vi "test15-StateBroadcast_Event.vi"(8 "error in (no error)":errorcluster, 11 "TestCase in":refnum<class "testcase-CSMGlobalLog.lvclass">) -> (0 "error out":errorcluster, 3 "TestCase out":refnum<class "testcase-CSMGlobalLog.lvclass">)   [LabVIEW 2017, in "testcase-CSMGlobalLog.lvclass"]
uses:
  testcase-CSMGlobalLog.lvclass
  testcase-CSMGlobalLog.lvclass/testcase-CSMGlobalLog.ctl
  src/user.lib/_NEVSTOP/Communicable State Machine(CSM)/_Support/Typedef/_CSM_GlobalLog_MSG.ctl
  src/user.lib/_NEVSTOP/Communicable State Machine(CSM)/_Support/Typedef/_CSM_Response Source Message.ctl
  src/user.lib/_NEVSTOP/Communicable State Machine(CSM)/_Support/Typedef/_CSM_GlobalLog_MSG_TYPE.ctl
  c0dc643a-0362-49fc-99f4-5251266ba5a0.vi
  src/user.lib/_NEVSTOP/Communicable State Machine(CSM)/_Support/GlobalEvent/GEvt-Generate with Rule Check.vi
  src/user.lib/_NEVSTOP/Communicable State Machine(CSM)/AdvanceAPI/CSM - Convert Error to Argument.vi
  src/user.lib/_NEVSTOP/Communicable State Machine(CSM)/AdvanceAPI/CSM - Make String Arguments Safe.vi
  src/user.lib/_NEVSTOP/Communicable State Machine(CSM)/AdvanceAPI/CSM - Keywords.vi
  src/user.lib/_NEVSTOP/Communicable State Machine(CSM)/_Support/GlobalEvent/Cache-GEvt Refs.vi
  src/user.lib/_NEVSTOP/Communicable State Machine(CSM)/_Support/GlobalEvent/LogFilter/LogFilter - Check.vi
  src/user.lib/_NEVSTOP/Communicable State Machine(CSM)/_Support/GlobalEvent/LogFilter/LogFilter.lvclass
  <vilib>/addons/_JKI Toolkits/VI Tester/TestCase.llb/TestCase.lvclass
  src/user.lib/_NEVSTOP/Communicable State Machine(CSM)/Communicable State Machine.lvlib
  C:/Program Files (x86)/National Instruments/LabVIEW 2017/vi.lib/addons/_JKI Toolkits/VI Tester/TestCase.llb/TestCase.lvclass
panel:
  out "String cache each loop":string
  out "error out 2":errorcluster
  out "Timed out":bool[](array[boolean])
  out "LoopCount":i32
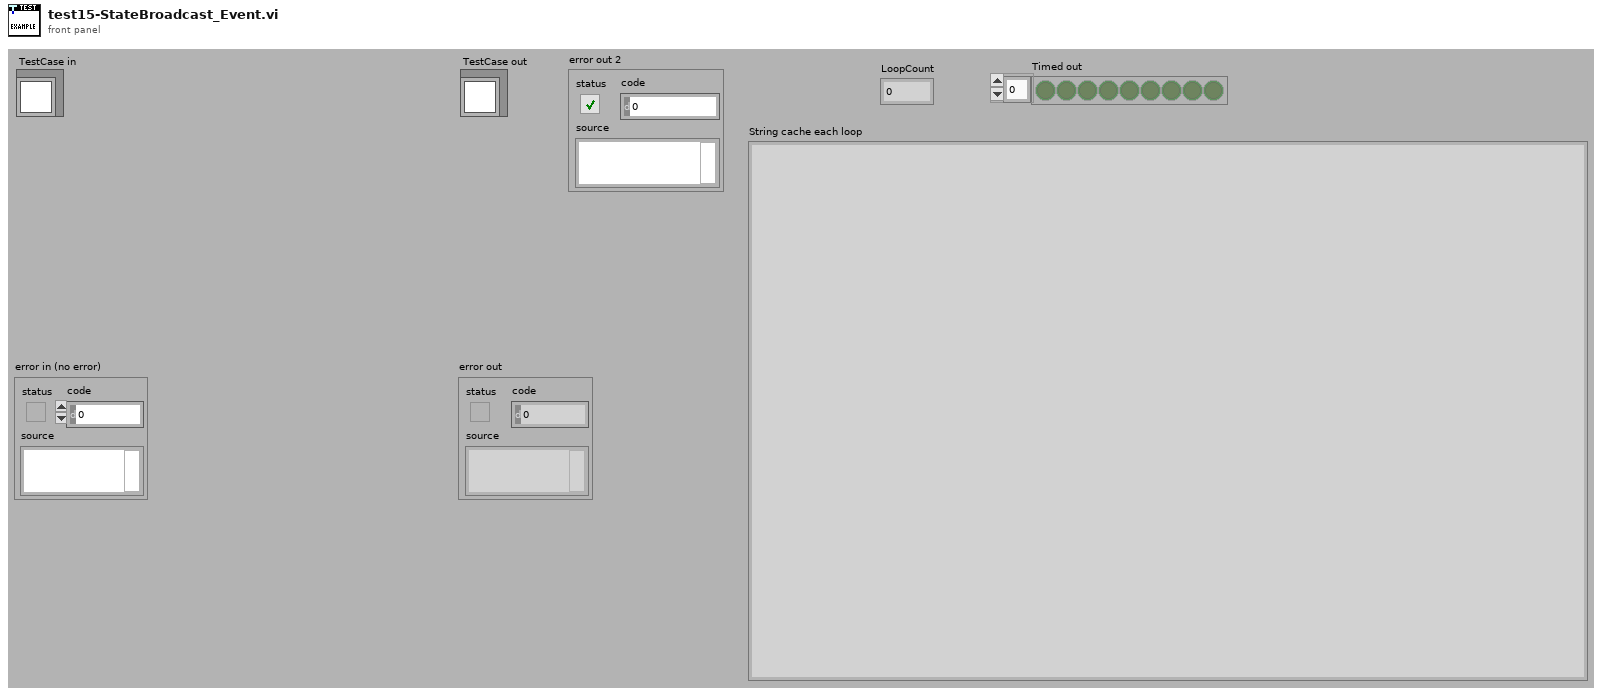
[diagram p1: front panel]
types:
  T1 = typedef "Communicable State Machine.lvlib/_CSM_GlobalLog_MSG.ctl" = cluster{"Name (\"\" to Use UUID)":string, "Current State":string, "Arguments":string, "Source Message":T2, "Source Module":string, "Complete(T)/Start(F)":bool, "LogType":T3, "Time Stamp":timestamp}
  T2 = typedef "Communicable State Machine.lvlib/_CSM_Response Source Message.ctl" = cluster{"‘State":string, "’Arguments":string, "’Error":errorcluster}
  T3 = typedef "Communicable State Machine.lvlib/_CSM_GlobalLog_MSG_TYPE.ctl" = enum16{"User Log", "State Change", "Status", "Interrupt", "Register", "Unregister", "Error Log", "Module Created", "Module Destroyed", "Async Message", "No-Rep Async Message", "Sync Message"}
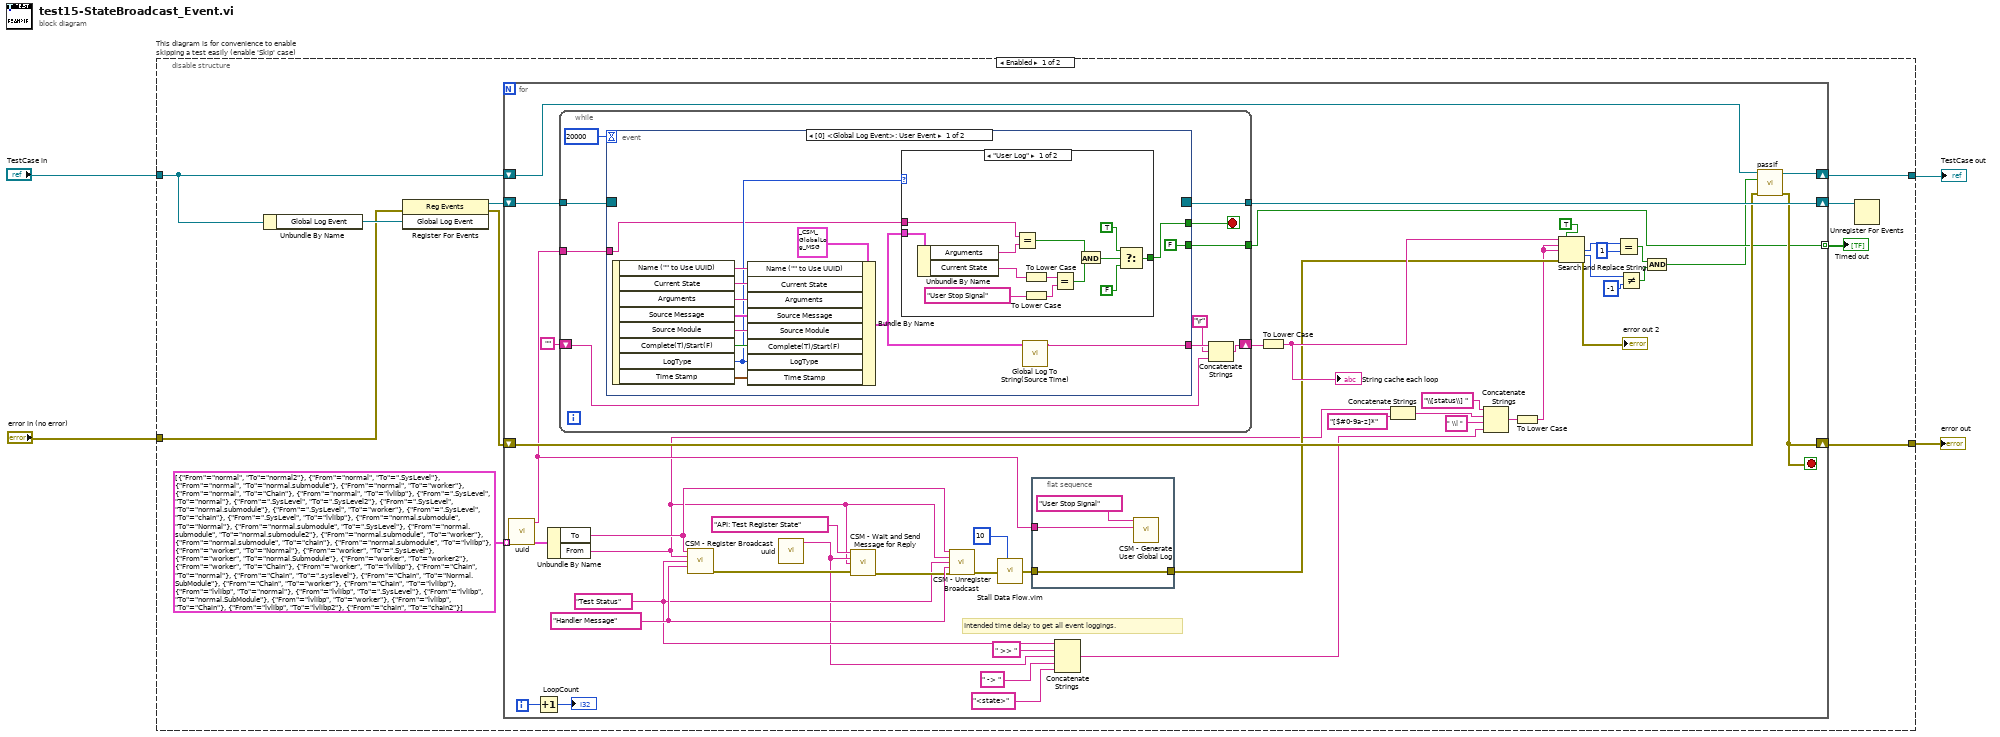
[diagram p0: block diagram]
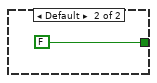
[diagram p2: hidden frame]
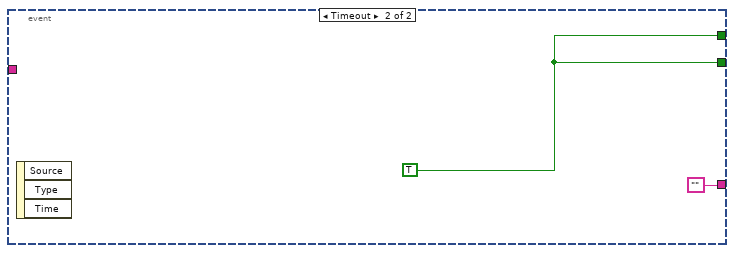
[diagram p3: hidden frame]
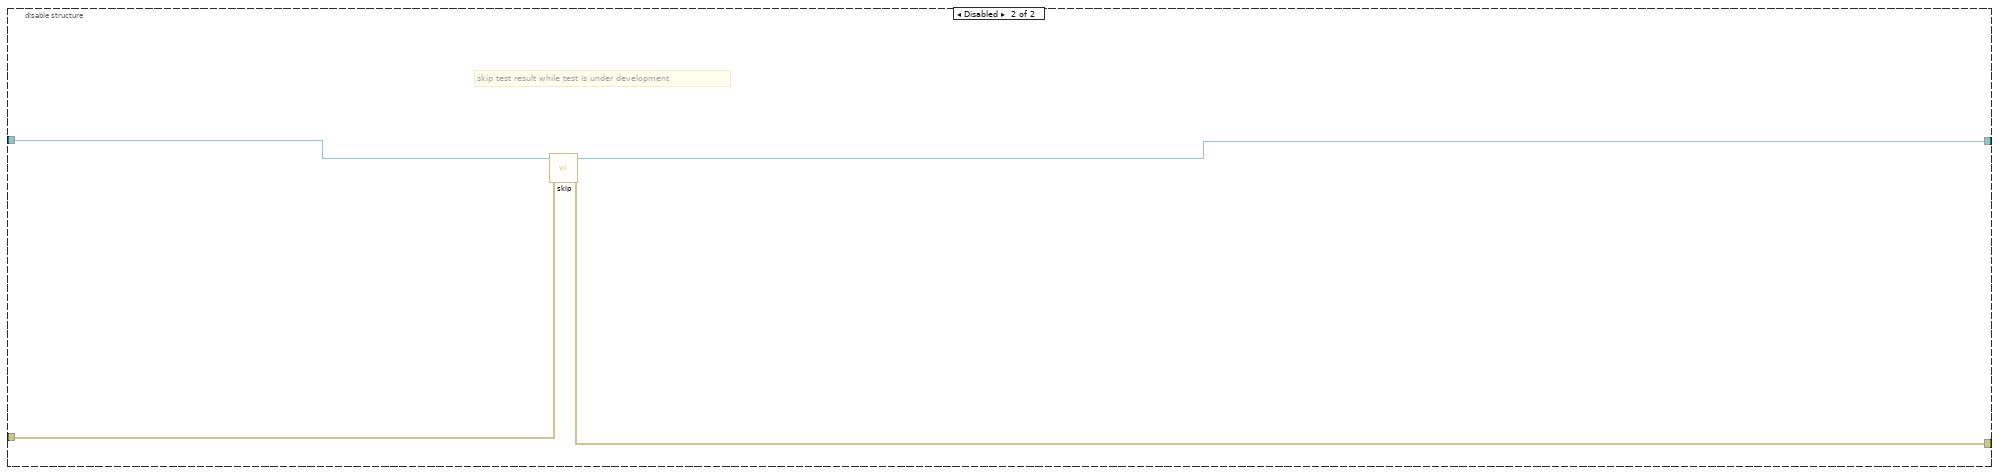
[diagram p4: hidden frame]
diagram:
  n1 = disable-structure "This diagram is for convenience to enable skipping a test easily (enable 'Skip' case)" shown="Enabled" {
    disable-tunnel: "TestCase in" -> [w9 w106]
    disable-tunnel: [w8 w104] -> w1
    disable-tunnel: [w7 w105] -> w3
    disable-tunnel: "error in (no error)" -> [w13 w103]
    frame Enabled {
      n2 = Unbundle By Name(w9) -> ("Global Log Event"=w14:refnum<user-event>)
      n3 = register-events(error in=w13, w14) -> (reference out=w12:refnum<event-registration>, error out=w10:errorcluster)  [unwired: 1 in]
      n4 = for {
        shift-right: [w58] -> w11
        shift-left: w12 -> [w59]
        shift-right: [w54] -> w7
        shift-left: w10 -> [w56]
        tunnel: cluster{"From":string, "To":string}[] [{"From"="normal", "To"="normal2"}, {"From"="normal", "To"=".SysLevel"}, {"From"="normal", "To"="normal.submodule"}, {"From"="normal", "To"="worker"}, {"From"="normal", "To"="Chain"}, {"From"="normal", "To"="lvlibp"}, {"From"=".SysLevel", "To"="normal"}, {"From"=".SysLevel", "To"=".SysLevel2"}, {"From"=".SysLevel", "To"="normal.submodule"}, {"From"=".SysLevel", "To"="worker"}, {"From"=".SysLevel", "To"="chain"}, {"From"=".SysLevel", "To"="lvlibp"}, {"From"="normal.submodule", "To"="Normal"}, {"From"="normal.submodule", "To"=".SysLevel"}, {"From"="normal.submodule", "To"="normal.submodule2"}, {"From"="normal.submodule", "To"="worker"}, {"From"="normal.submodule", "To"="chain"}, {"From"="normal.submodule", "To"="lvlibp"}, {"From"="worker", "To"="Normal"}, {"From"="worker", "To"=".SysLevel"}, {"From"="worker", "To"="normal.Submodule"}, {"From"="worker", "To"="worker2"}, {"From"="worker", "To"="Chain"}, {"From"="worker", "To"="lvlibp"}, {"From"="Chain", "To"="normal"}, {"From"="Chain", "To"=".syslevel"}, {"From"="Chain", "To"="Normal.SubModule"}, {"From"="Chain", "To"="worker"}, {"From"="Chain", "To"="lvlibp"}, {"From"="lvlibp", "To"="normal"}, {"From"="lvlibp", "To"=".SysLevel"}, {"From"="lvlibp", "To"="normal.SubModule"}, {"From"="lvlibp", "To"="worker"}, {"From"="lvlibp", "To"="Chain"}, {"From"="lvlibp", "To"="lvlibp2"}, {"From"="chain", "To"="chain2"}] -> [w31] mode=indexing
        shift-right: [w57] -> w8
        shift-left: w9 -> [w53]
        tunnel: [w37] -> w5 mode=indexing
        i -> [w42]
        stop <- w54 stop-if-true
        w36 = "Handler Message" ("API (If \"\", Same as Trigger)")
        w27 = "Test Status" ("Trigger")
        # "Intended time delay to get all event loggings."
        n5 = call "uuid.vi"() -> ("UUID"=w43:string)  [unwired: 11 in]
        n6 = Increment(x=w42) -> (x+1=→"LoopCount":i32)
        n7 = Unbundle By Name(w31) -> ("To"=w18:string, "From"=w17:string)
        n8 = while {
          tunnel: w59 -> [w72]
          tunnel: [w71] -> w58
          shift-right: [w63] -> w38
          shift-left: "" -> [w66]
          tunnel: w43 -> [w68]
          tunnel: [w67] -> w37
          stop <- w70 stop-if-true
          n9 = event shown="[0] <Global Log Event>: User Event" {
            selector: w72 -> [_ _]
            dyn-events: [_ _] -> w71
            timeout: 20000 -> [_ _]
            tunnel: [w73 ""] -> w65
            tunnel: [w75 w102] -> w70
            tunnel: w68 -> [w76 _]
            tunnel: [FALSE ("Stop") w102] -> w67
            event User Event {
              n10 = event-data() -> ("Name (\"\" to Use UUID)"=w85:string, "Current State"=w84:string, "Arguments"=w83:string, "Source Message"=w82:T2, "Source Module"=w81:string, "Complete(T)/Start(F)"=w80:bool, "LogType"=w77:T3, "Time Stamp"=w79:timestamp)  [unwired: 1 in]
              n11 = Bundle By Name(cluster=T1 {"Name (\"\" to Use UUID)"="", "Current State"="", "Arguments"="", "Source Message"={"‘State"="", "’Arguments"="", "’Error"={"status"=FALSE, "code"=0, "source"=""}}, "Source Module"="", "Complete(T)/Start(F)"=FALSE, "LogType"=enum."State Change", "Time Stamp"=timestamp(0 s since 1904-01-01)} ("Cross CSM Data"), "Name (\"\" to Use UUID)"=w85, "Current State"=w84, "Arguments"=w83, "Source Message"=w82, "Source Module"=w81, "Complete(T)/Start(F)"=w80, "LogType"=w77, "Time Stamp"=w79) -> (w74:T1)
              n12 = case shown="\"User Log\"" w77 {
                tunnel: w74 -> [w99 _]
                tunnel: w76 -> [w98 _]
                tunnel: [w87 FALSE] -> w75
                frame "User Log" {
                  n13 = Unbundle By Name(w99) -> ("Arguments"=w97:string, "Current State"=w96:string)
                  n14 = Equal?(x=w98, y=w97) -> (x = y?=w91:bool)
                  n15 = To Lower Case(string=w96) -> (all lower case string=w95:string)
                  n16 = To Lower Case(string="User Stop Signal" ("Log")) -> (all lower case string=w93:string)
                  n17 = Equal?(x=w95, y=w93) -> (x = y?=w92:bool)
                  n18 = And(x=w91, y=w92) -> (x .and. y?=w90:bool)
                  n19 = Select(t=TRUE, s=w90, f=FALSE) -> (s? t:f=w87:bool)
                }
                frame Default {
                }
              }
              n20 = call "Global Log To String(Source Time).vi"("Log"=w74) -> ("Log String"=w73:string)  [unwired: 9 in]
            }
            event Timeout {
              w102 = TRUE ("Stop")
              n21 = event-data() -> ()  [unwired: 1 in, 3 out]
            }
          }
          n22 = Concatenate Strings(w65, "\r", w66) -> (w63:string)
        }
        n23 = call "CSM - Register Broadcast.vi"("CSM Name(Empty for Broadcast Event)"=w18, "Source CSM Name (* as Default)"=w17, "Trigger"=w27, "API (If \"\", Same as Trigger)"=w36) -> ("error out"=w33:errorcluster)  [unwired: 10 in, 1 out]
        n24 = call "uuid.vi"() -> ("UUID"=w26:string)  [unwired: 11 in]
        n25 = call "CSM - Wait and Send Message for Reply.vi"("State"="API: Test Register State", "Arguments (\"\")"=w26, "Target Module"=w17, "Error In (No Error)"=w33) -> ("error out"=w34:errorcluster)  [unwired: 8 in, 3 out]
        n26 = call "CSM - Unregister Broadcast.vi"("CSM Name(Empty for Broadcast Event)"=w18, "Source CSM Name (* as Default)"=w17, "Trigger"=w27, "API (\"*\" as Default)"=w36, "Error In"=w34) -> ("error out"=w32:errorcluster)  [unwired: 9 in, 1 out]
        n27 = call "Stall Data Flow.vim"("value in"=w32, "milliseconds to wait"=u32 10) -> ("value out"=w44:errorcluster)  [unwired: 1 out]
        n28 = flat-sequence {
          tunnel: w43 -> [w61]
          tunnel: w44 -> [w60]
          tunnel: [w60] -> w39
          frame #0 {
            n29 = call "CSM - Generate User Global Log.vi"("Arguments"=w61, "Log"="User Stop Signal") -> ()  [unwired: 9 in, 1 out]
          }
        }
        n30 = Concatenate Strings(w27, " >> " ("string"), w26, " -> " ("string"), "<state>" ("search string")) -> (w16:string)
        n31 = To Lower Case(string=w38) -> (all lower case string=w40:string)
        "String cache each loop" <- w40
        n32 = Concatenate Strings(w17, "[$#0-9a-z]*" ("string")) -> (w19:string)
        n33 = Concatenate Strings("\\[status\\] " ("regular expression"), w19, " \\| " ("string"), w16) -> (w22:string)
        n34 = To Lower Case(string=w22) -> (all lower case string=w15:string)
        n35 = Search and Replace String(replace all?=TRUE ("replace all? (F)"), input string=w40, search string=w15, replace string=w15, error in=w39) -> (number of replacements=w49:i32, offset past replacement=w50:i32, error out=→"error out 2":errorcluster)  [unwired: 3 in, 1 out]
        n36 = Equal?(x=w49, y=1) -> (x = y?=w51:bool)
        n37 = Not Equal?(x=w50, y=-1) -> (x != y?=w52:bool)
        n38 = And(x=w51, y=w52) -> (x .and. y?=w25:bool)
        n39 = call-dynamic "passIf.vi"("error in (no error)"=w56, "pass"=w25, "TestCase in"=w53) -> ("error out"=w54:errorcluster, "TestCase out"=w57:refnum<class "testcase-CSMGlobalLog.lvclass">)  [unwired: 7 in]
      }
      "Timed out" <- w5
      n40 = Unregister For Events(event registration refnum=w11) -> ()  [unwired: 1 in, 1 out]
    }
    frame Disabled {
      # "skip test result while test is under development"
      n41 = call <vilib>:"skip.vi"("error in (no error)"=w103, "TestCase in"=w106) -> ("error out"=w105:errorcluster, "TestCase out"=w104:refnum<class "testcase-CSMGlobalLog.lvclass">)  [unwired: 8 in]
    }
  }
  "error out" <- w3
  "TestCase out" <- w1
